vi "GetEncoderValues.vi"(8 "error in":errorcluster) -> (0 "error out":errorcluster, 2 "RightDistance":dbl, 3 "LeftDistance":dbl)   [LabVIEW 2016]
uses:
  Robot Global Data.vi
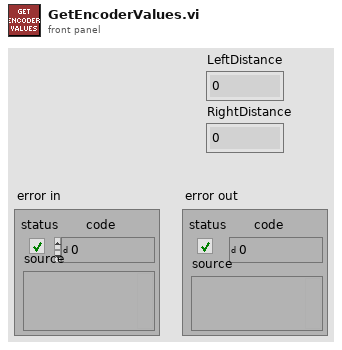
[diagram p1: front panel]
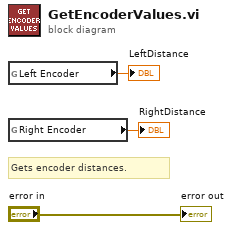
[diagram p0: block diagram]
diagram:
  # "Gets encoder distances."
  n1 = global read "Robot Global Data.vi" "Left Encoder"() -> (→"LeftDistance":dbl)
  n2 = global read "Robot Global Data.vi" "Right Encoder"() -> (→"RightDistance":dbl)
  "error out" <- "error in"
